vi "Enter Serial Number Prompt1.vi"(1 "InputArray":string[](array[string]), 2 "data storage path":path) -> (0 "OutputArray":string[](array[string]))   [LabVIEW 2021]
panel:
  in  "aging spec2 (ppb/day)":string
  in  "Engr Test":bool
  in  "Position No":string
  in  "System No":string
  in  "Rack No":string
  in  "Age Temp":string
  in  "Nominal":string
  in  "aging spec (ppm)":string
  in  "Days for spec":string
  in  "Gate time":string
  in  "Fixture Serial Number":string
  in  "Card Serial Number":string
  in  "Serial  Number":string
  in  "Part Number":string
  in  "Work Order Number":string
  out "Title":string
  in  "OK":bool
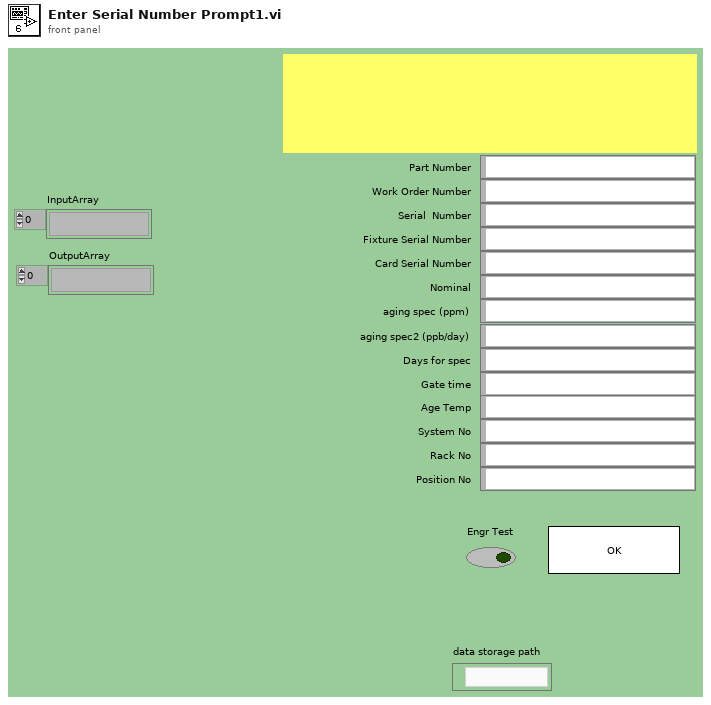
[diagram p1: front panel]
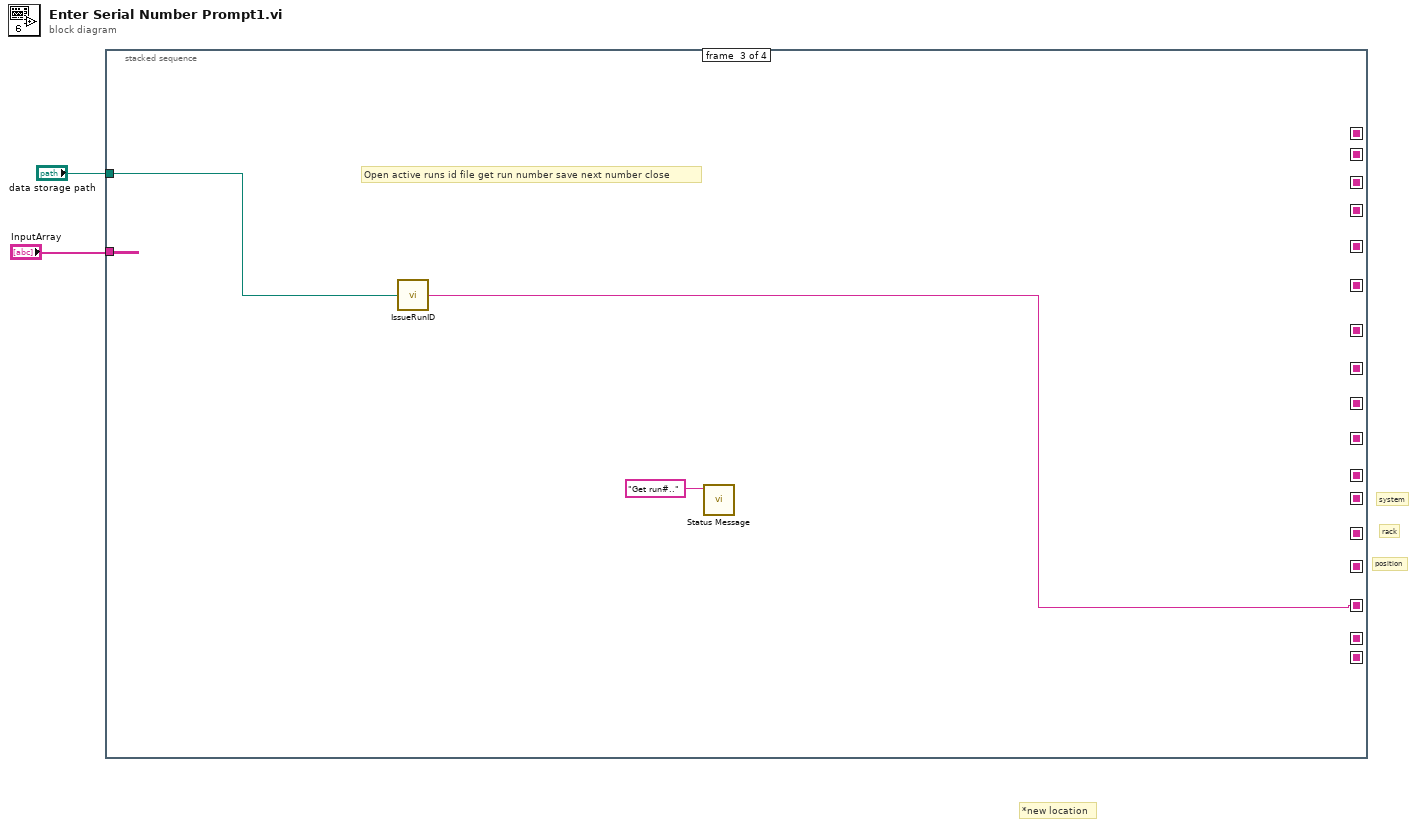
[diagram p0: block diagram]
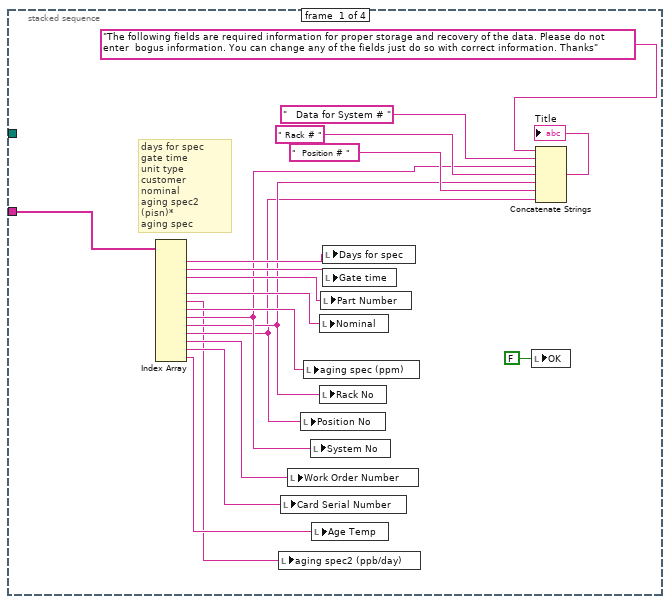
[diagram p2: hidden frame]
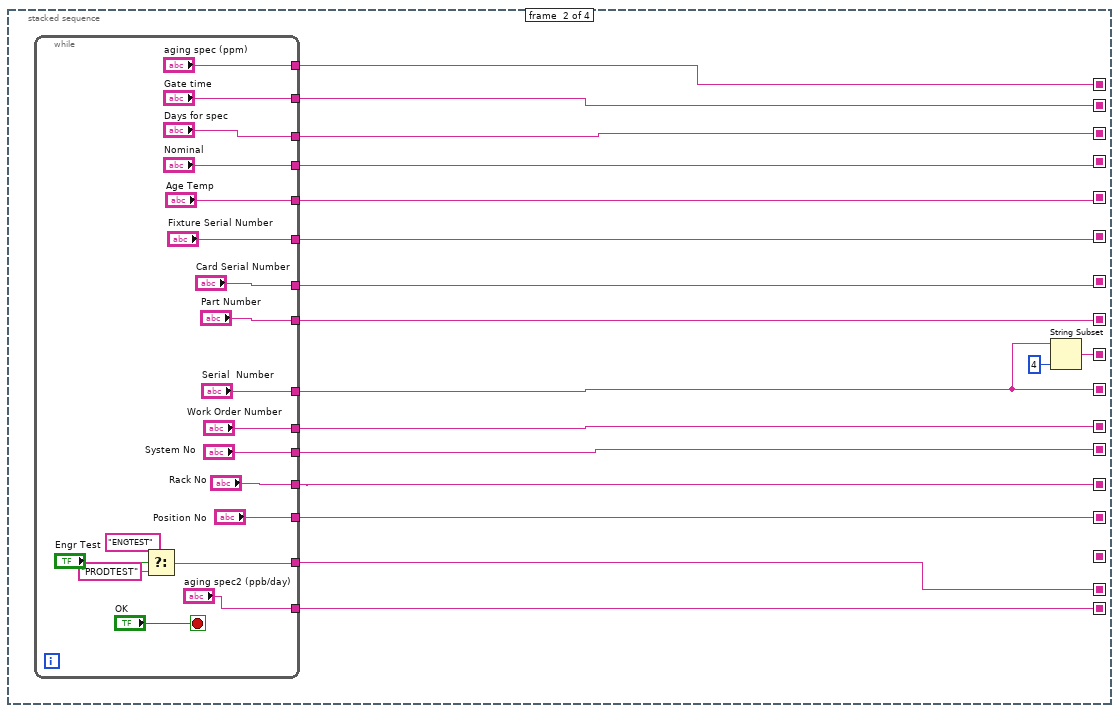
[diagram p3: hidden frame]
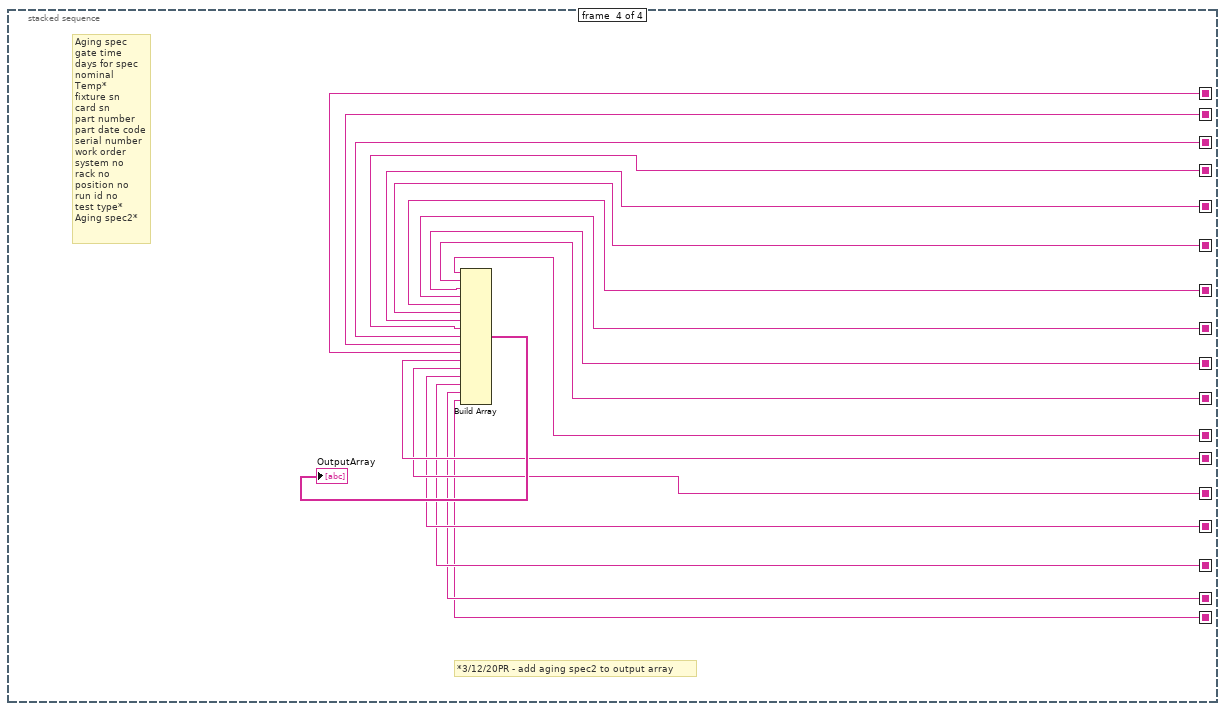
[diagram p4: hidden frame]
diagram:
  # "*new location"
  # "position"
  # "rack"
  # "system"
  n1 = stacked-sequence {
    seq-local: [_ w38 _ _] -> [_ _ _ w68]
    seq-local: [_ w37 _ _] -> [_ _ _ w69]
    seq-local: [_ w36 _ _] -> [_ _ _ w70]
    seq-local: [_ w35 _ _] -> [_ _ _ w71]
    seq-local: [_ w34 _ _] -> [_ _ _ w72]
    seq-local: [_ w33 _ _] -> [_ _ _ w73]
    seq-local: [_ w32 _ _] -> [_ _ _ w74]
    seq-local: [_ w31 _ _] -> [_ _ _ w75]
    seq-local: [_ w25 _ _] -> [_ _ _ w76]
    seq-local: [_ w23 _ _] -> [_ _ _ w77]
    seq-local: [_ w30 _ _] -> [_ _ _ w78]
    seq-local: [_ w29 _ _] -> [_ _ _ w66]
    seq-local: [_ w28 _ _] -> [_ _ _ w65]
    seq-local: [_ w27 _ _] -> [_ _ _ w64]
    seq-local: [_ _ w59 _] -> [_ _ _ w63]
    seq-local: [_ w26 _ _] -> [_ _ _ w62]
    seq-local: [_ w22 _ _] -> [_ _ _ w61]
    tunnel: "InputArray" -> [w12 _ _ _]
    tunnel: "data storage path" -> [_ _ w60 _]
    frame #0 {
      # "days for spec\ngate time\nunit type\ncustomer\nnominal\naging spec2 (pisn)*\naging spec"
      n2 = Index Array(array=w12) -> (element #1=w17:string, element #2=w16:string, element #3=w15:string, element #5=w14:string, element #6=w3:string, element #7=w13:string, element #8=w9:string, element #9=w8:string, element #10=w7:string, element #11=w6:string, element #12=w5:string, element #13=w4:string)  [unwired: 13 in, 1 out]
      n3 = local write "aging spec2 (ppb/day)"(w3) -> ()
      n4 = local write "Card Serial Number"(w5) -> ()
      n5 = local write "Work Order Number"(w6) -> ()
      n6 = local write "Position No"(w7) -> ()
      n7 = local write "aging spec (ppm)"(w13) -> ()
      n8 = local write "System No"(w9) -> ()
      n9 = local write "Age Temp"(w4) -> ()
      n10 = local write "Nominal"(w14) -> ()
      n11 = local write "Rack No"(w8) -> ()
      n12 = local write "Part Number"(w15) -> ()
      n13 = local write "Days for spec"(w17) -> ()
      n14 = local write "Gate time"(w16) -> ()
      n15 = local write "OK"(FALSE ("OK")) -> ()
      n16 = Concatenate Strings("The following fields are required information for proper storage and recovery of the data. Please do not enter  bogus information. You can change any of the fields just do so with correct information. Thanks", "   Data for System # ", w9, " Rack # ", w8, "  Position # ", w7) -> (→"Title":string)
    }
    frame #1 {
      n17 = while {
        tunnel: ["Work Order Number"] -> w30
        tunnel: ["Serial  Number"] -> w23
        tunnel: ["Fixture Serial Number"] -> w33
        tunnel: ["Card Serial Number"] -> w32
        tunnel: ["Part Number"] -> w31
        tunnel: ["aging spec (ppm)"] -> w38
        tunnel: ["Gate time"] -> w37
        tunnel: ["Days for spec"] -> w36
        tunnel: ["Nominal"] -> w35
        tunnel: ["Age Temp"] -> w34
        tunnel: ["System No"] -> w29
        tunnel: ["Rack No"] -> w28
        tunnel: ["Position No"] -> w27
        tunnel: [w41] -> w26
        tunnel: ["aging spec2 (ppb/day)"] -> w22
        stop <- "OK" stop-if-true
        n18 = Select(t="ENGTEST", s="Engr Test", f="PRODTEST") -> (s? t:f=w41:string)
      }
      n19 = String Subset(string=w23, length (rest)=4 ("length (rest)")) -> (substring=w25:string)  [unwired: 1 in]
    }
    frame #2 {
      # "Open active runs id file get run number save next number close"
      n20 = call "IssueRunID.vi"("data storage path"=w60) -> ("Run ID"=w59:string)
      n21 = call "Status Message.vi"(11:"Get run#..") -> ()  [unwired: 11 in]
    }
    frame #3 {
      # "*3/12/20PR - add aging spec2 to output array"
      # "Aging spec\ngate time\ndays for spec\nnominal\nTemp*\nfixture sn\ncard sn\npart number\npart date code\nserial number\nwork order\nsystem no\nrack no\nposition no\nrun id no\ntest type*\nAging spec2*"
      n22 = Build Array(w78, w77, w76, w75, w74, w73, w72, w71, w70, w69, w68, w66, w65, w64, w63, w62, w61) -> (→"OutputArray":string[])
    }
  }
